vi "Midterm.vi"() -> ()   [LabVIEW 2019]
uses:
  <vilib>/httpClient/LabVIEWHTTPClient.lvlib
panel:
  out "element":string
  out "body":string
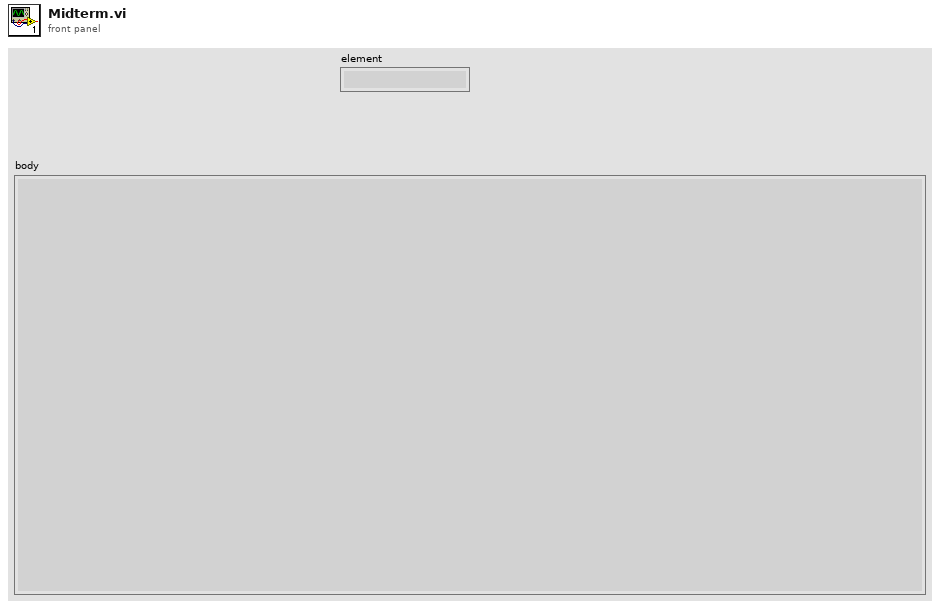
[diagram p1: front panel]
types:
  T1 = cluster{"menu-id":string, "data":cluster{"Breakfast":cluster{"BREAKFAST ENTREE":string[]}}}
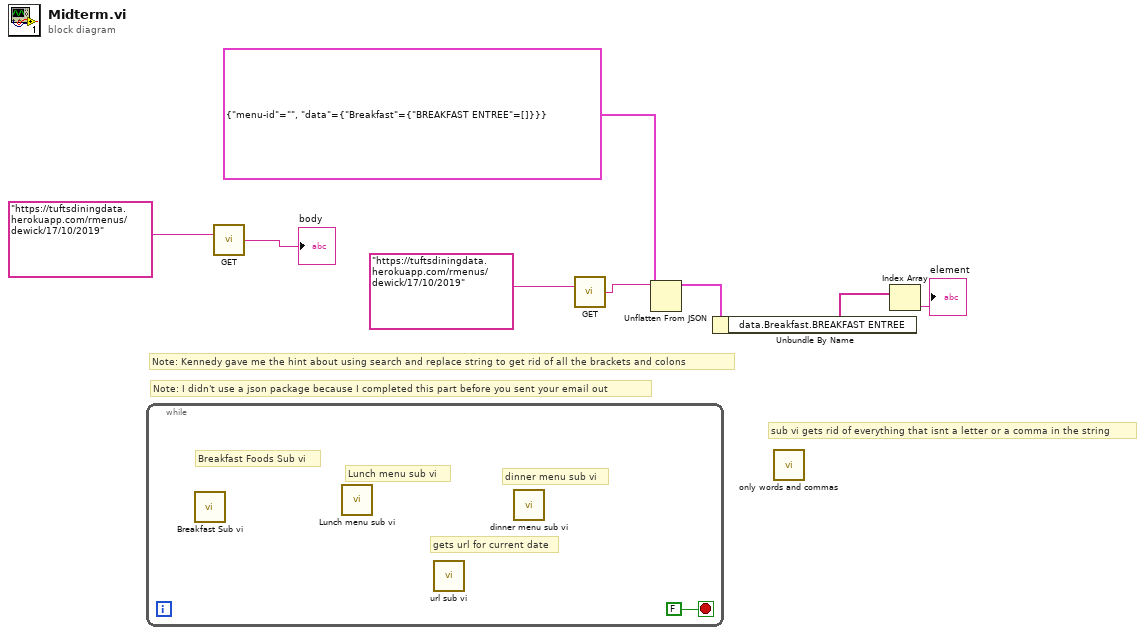
[diagram p0: block diagram]
diagram:
  # "Note: I didn't use a json package because I completed this part before you sent your email out"
  # "sub vi gets rid of everything that isnt a letter or a comma in the string"
  # "Note: Kennedy gave me the hint about using search and replace string to get rid of all the brackets and colons"
  n1 = while {
    stop <- FALSE stop-if-true
    # "gets url for current date"
    # "dinner menu sub vi"
    # "Lunch menu sub vi"
    # "Breakfast Foods Sub vi"
    n2 = call "Breakfast Sub vi.vi"() -> ()  [unwired: 8 in, 4 out]
    n3 = call "Lunch menu sub vi.vi"() -> ()  [unwired: 12 in]
    n4 = call "url sub vi.vi"() -> ()  [unwired: 11 in, 1 out]
    n5 = call "dinner menu sub vi.vi"() -> ()  [unwired: 12 in]
  }
  n6 = call <vilib>:"GET.vi"("url"="https://tuftsdiningdata.herokuapp.com/rmenus/dewick/17/10/2019") -> ("body"=→"body":string)  [unwired: 11 in, 3 out]
  n7 = call <vilib>:"GET.vi"("url"="https://tuftsdiningdata.herokuapp.com/rmenus/dewick/17/10/2019") -> ("body"=w5:string)  [unwired: 11 in, 3 out]
  n8 = Unflatten From JSON(JSON string=w5, type and defaults=T1 {"menu-id"="", "data"={"Breakfast"={"BREAKFAST ENTREE"=[]}}}) -> (value=w3:T1)  [unwired: 5 in, 1 out]
  n9 = Unbundle By Name(w3) -> ("data.Breakfast.BREAKFAST ENTREE"=w2:string[])
  n10 = call "only words and commas.vi"() -> ()  [unwired: 11 in, 1 out]
  n11 = Index Array(array=w2) -> (element=→"element":string)  [unwired: 1 in]
